vi "RealSense_HelloWorld_PointCloud.vi"() -> ()   [LabVIEW 2016]
doc: "Simple Demo showing how to connect a RealSense Camera to stream COLOR and DEPTH from the stereo camera of a D4xx series camera."
uses:
  <vilib>/Utility/miscctls.llb/LV3DPointTypeDef.ctl
  <vilib>/Utility/miscctls.llb/LVRGBAColorTypeDef.ctl
  <vilib>/picture/3D Picture Control/Object/Create Object (name).vi
  libRealSense3.lvlib
  <vilib>/picture/3D Picture Control/NI_3D Picture Control.lvlib
panel:
  in  "Display tab":T1(tab)
  out "Found \nRealSense":bool=TRUE
  out "height":i32=720
  out "width":i32=1280
  out "init results":T2={"camera name"="Intel RealSense 415", "camera S/N"="725112060291", "F/W"="05.08.08.00", "Sensor name"="Stereo Module", "api_version"=20801, "rscontext"=1827613840, "device_list"=610165840, "device count"=2, "Dev out"=1824884112, "sensor_list"=1824885136, "sensor count"=2, "Sensor out"=609327328}
  in  "Select Resolution":u16(ring)=27 items=["424 x 240 @6fps", "424 x 240 @15fps", "424 x 240 @30fps", "424 x 240 @60fps", "424 x 240 @90fps", "480 x 270 @6fps", "480 x 270 @15fps", "480 x 270 @30fps", "480 x 270 @60fps", "480 x 270 @90fps", "640 x 360 @6fps", "640 x 360 @15fps", "640 x 360 @30fps", "640 x 360 @60fps", "640 x 360 @90fps", "640 x 480 @6fps", "640 x 480 @15fps", "640 x 480 @30fps", "640 x 480 @60fps", "640 x 480 @90fps", "848 x 480 @6fps", "848 x 480 @15fps", "848 x 480 @30fps", "848 x 480 @60fps", "848 x 480 @90fps", "1280 x 720 @6fps", "1280 x 720 @15fps", "1280 x 720 @30fps"]
  in  "Sensor index":i32
  in  "Device index":i32
  out "L-R Baseline, mm":sgl=54.83181
  out "fy":sgl=952.6064 format="%#_5g"
  out "fx":sgl=952.6064 format="%#_5g"
  out "ppy":sgl=370.69974 format="%#_5g"
  out "ppx":sgl=634.5728 format="%#_5g"
  in  "Exposure,us":sgl=33000.0
  in  "Autoexposure":bool=TRUE
  in  "Depth Presets":T3(ring)=enum."Face2"
  in  "Color Presets":T4(ring)=enum."DS410 (DS5a) 4"
  in  "Laser on/off":bool=TRUE
  in  "Gain(16-248)":sgl=16.0 min=16 max=248
  in  "Update Presets":bool
  in  "Laser \nPower (mW)":dbl(slide)=155.72448 min=0.0 max=360.0 scale=0.36..360.0
  in  "Range Scale":enum16{"200m", "100m", "60m", "6m", "2m", "1m"}(ring)=enum."6m"
  out "RGB image":picture
  out "Depth map":sgl[][](graph)
  out "3D Picture":refnum<vi>(3d-picture)
  out "init error":string="No Error\rNo Error\rNo Error\rNo Error\rNo Error\rNo Error\rNo Error\rNo Error\rNo Error\rNo Error\rNo Error"
  out "Capture2 error":string="No Error"
  out "Start Error":string="No Error\rNo Error\rNo Error"
  out "Config error":string="No Error\rNo Error"
  out "Capture1 Error":string="No Error"
  out "Close Error":string="No Error\rNo Error\rNo Error\rNo Error"
  out "release frame error":string="No Error"
  out "iteration":i32=57
  in  "stop":bool=TRUE
  # "RealSense Hello World: PointCloud"
  # "This demo shows how to connect a RealSense D4xx Stereo Depth Camera, and display the textured PointCloud."
  # "Note; When you change Depth Preset you need to stop and restart for the HDAD settings to take effect.\n\nTry the Color preset called \"Remove IR2\". It will remove the laser projector from the RGB 1280x720 image."
  # "INTRINSICS & EXTRINSICS"
  # "SELECT THE RESOLUTION"
  # "DEPTH MAP"
  # "COLOR"
  # "Changes Color scale for Depth Map."
  # "20-1660000"
  # "3D POINTCLOUD"
  # "Rotate: Drag image\nMove X-Y: HOLD DOWN CTRL while dragging.\nZoom: SHIFT while dragging."
  # "ERRORS"
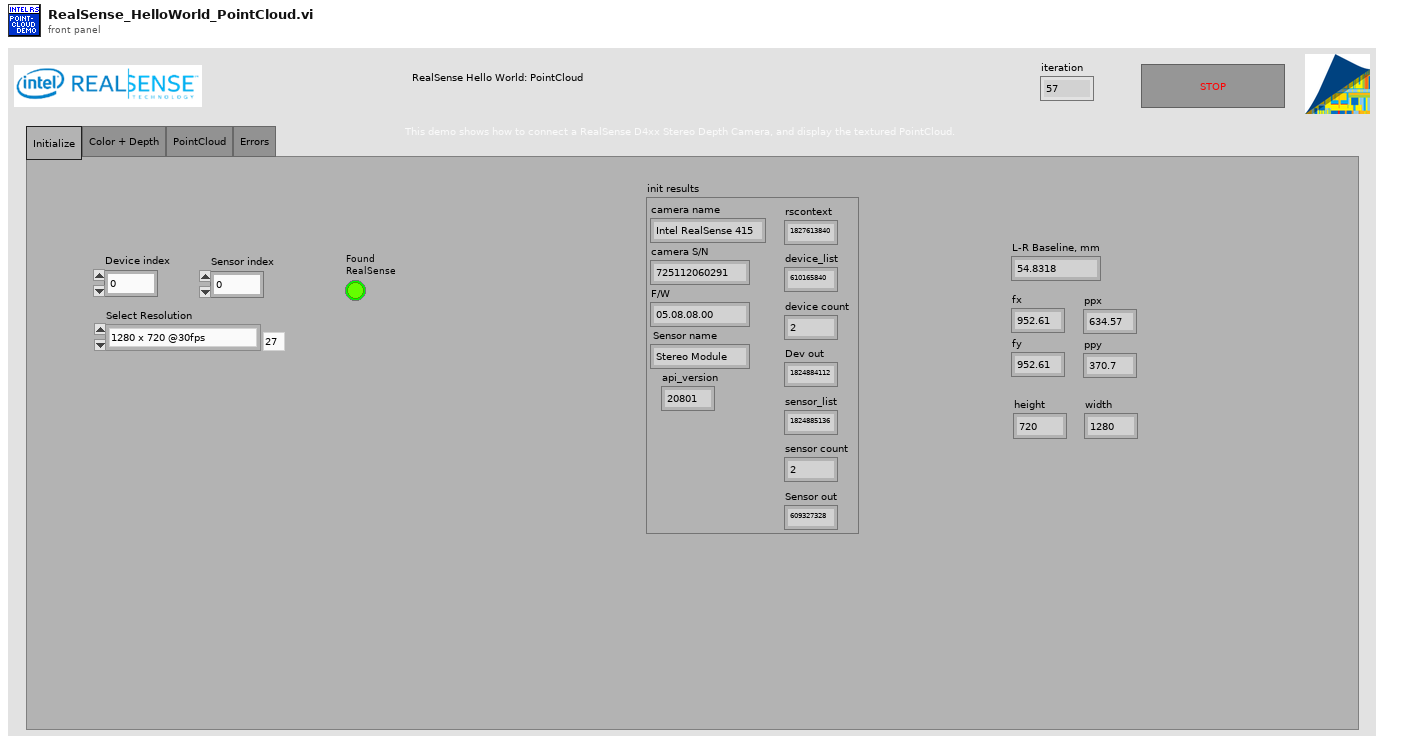
[diagram p1: front panel]
types:
  T1 = enum32{"Initialize", "Color + Depth", "PointCloud", "Errors"}
  T2 = cluster{"camera name":string, "camera S/N":string, "F/W":string, "Sensor name":string, "api_version":i32, "rscontext":u64, "device_list":u64, "device count":i32, "Dev out":u64, "sensor_list":u64, "sensor count":i32, "Sensor out":u64}
  T3 = enum16{"Custom", "Original", "New Depth 1", "New Depth 2", "Depth Active 1", "Active 3D Scan", "Active Short A", "Active Short C", "Face", "Face2", "Best Box", "High Density", "Medium Density", "High Accuracy", "Hand", "Short Range", "Flat wall", "Load .JSON", "Load .JSON2"}
  T4 = enum16{"Custom", "RS400 (DS5p)", "RS400 (DS5p) 2", "RS400 (DS5p) 3", "RS400 (DS5p) 4", "RS400 (DS5p) 5", "RS410 (DS5a)", "RS410 (DS5a) 2", "DS410 (DS5a) 3", "DS410 (DS5a) 4", "DS410+IR", "DS5LR", "DS5LR-2", "DS5LR no pattern", "RS410 Remove IR", "RS410 Remove IR 2", "DS5micro", "D435"}
  T5 = cluster{"width":i32, "height":i32, "fps":i32, "Profile":u64, "ppx":sgl, "ppy":sgl, "fx":sgl, "fy":sgl, "model":u32}
  T6 = enum16{"Overall", "Per Primitive", "Per Vertex", "Binding Off"}
  T7 = enum16{"Points", "Lines", "Line Strip", "Line Loop", "Triangles", "Triangle Strip", "Triangle Fan", "Quads", "Quad Strip", "Polygon"}
  T8 = enum16{"Depth", "Color (ext.)", "Color (left) ", "IR Left", "IR Right", "IR Left (Y16)", "IR Right (Y16)"}
  T9 = cluster{"R":dbl, "G":dbl, "B":dbl, "Alpha":dbl}[]
  T10 = typedef "LVRGBAColorTypeDef.ctl" = cluster{"Red":sgl, "Green":sgl, "Blue":sgl, "Alpha":sgl}
  T11 = typedef "LV3DPointTypeDef.ctl" = cluster{"X":sgl, "Y":sgl, "Z":sgl}
  T12 = cluster{"Alpha":sgl, "Blue":sgl, "Green":sgl, "Red":sgl}
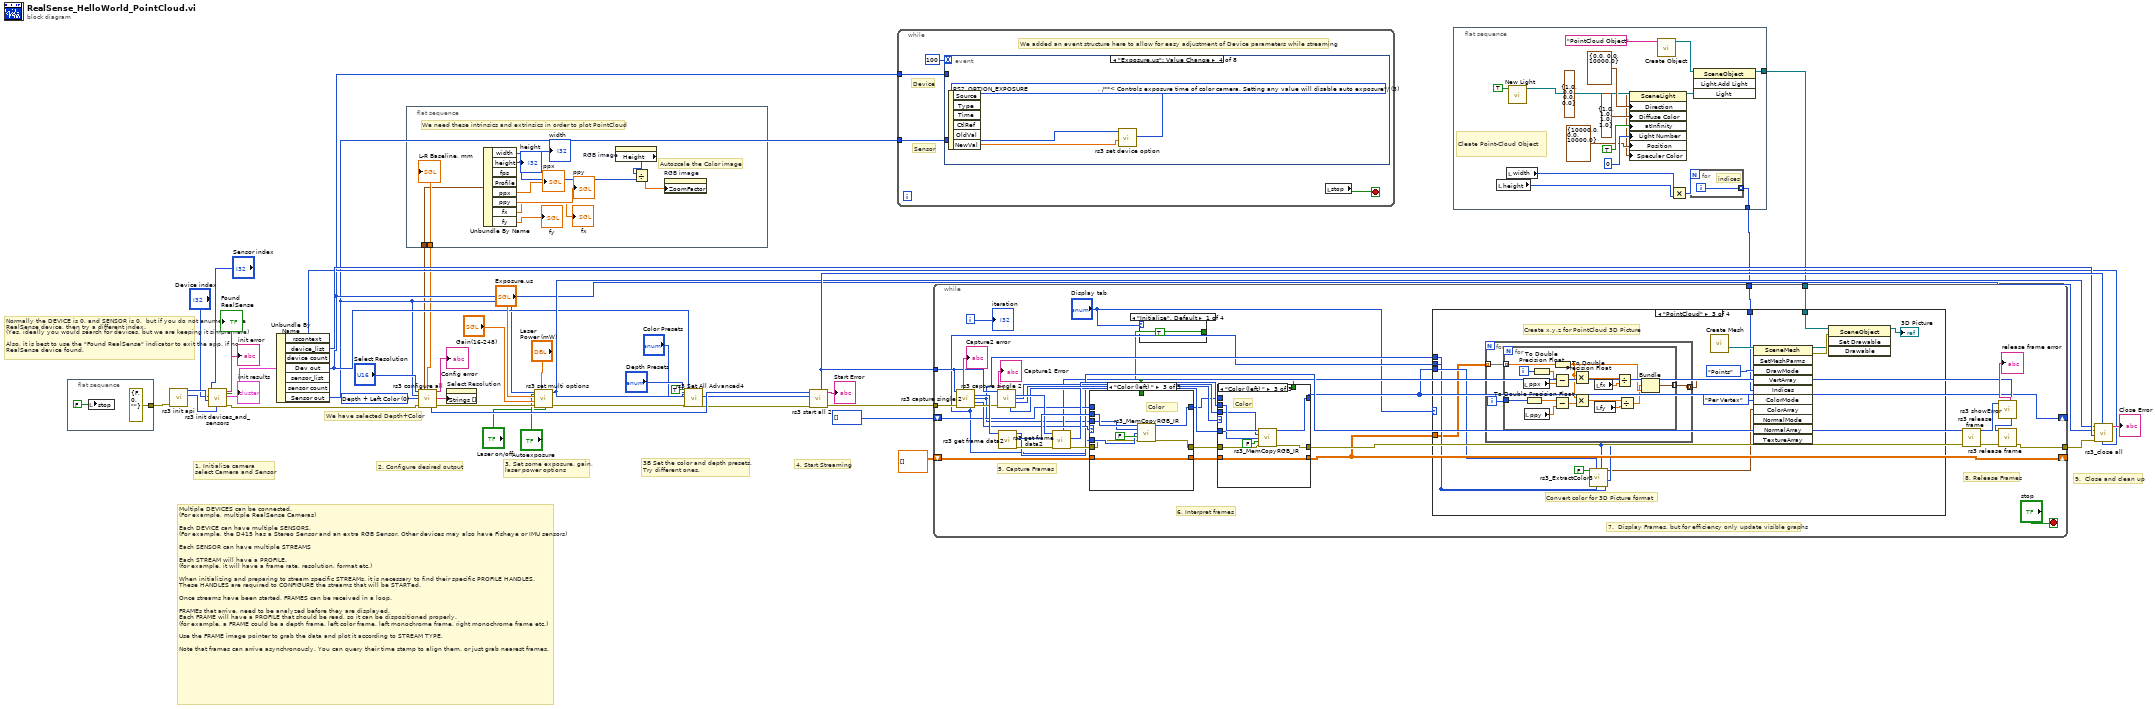
[diagram p0: block diagram]
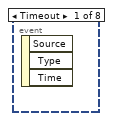
[diagram p2: hidden frame]
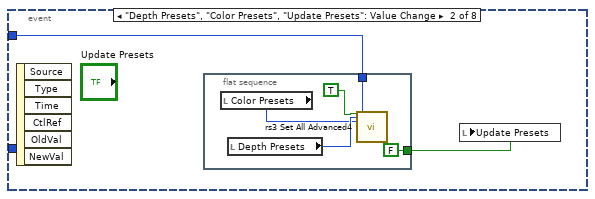
[diagram p3: hidden frame]
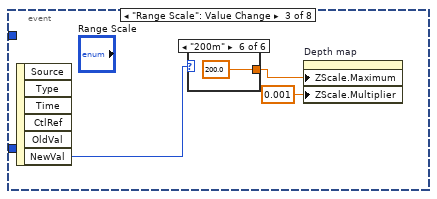
[diagram p4: hidden frame]
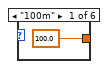
[diagram p5: hidden frame]
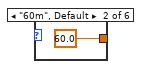
[diagram p6: hidden frame]
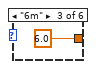
[diagram p7: hidden frame]
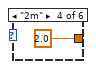
[diagram p8: hidden frame]
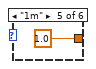
[diagram p9: hidden frame]
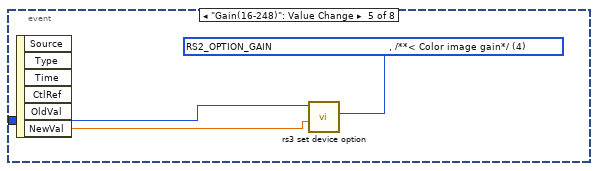
[diagram p10: hidden frame]
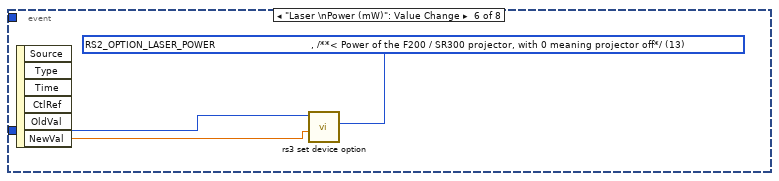
[diagram p11: hidden frame]
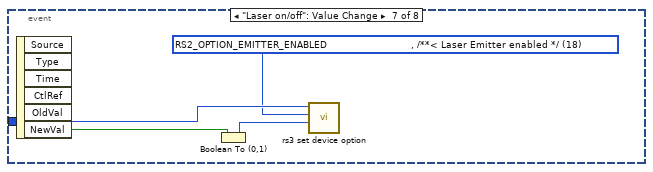
[diagram p12: hidden frame]
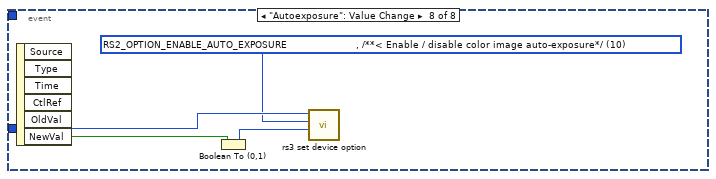
[diagram p13: hidden frame]
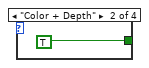
[diagram p14: hidden frame]
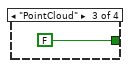
[diagram p15: hidden frame]
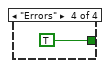
[diagram p16: hidden frame]
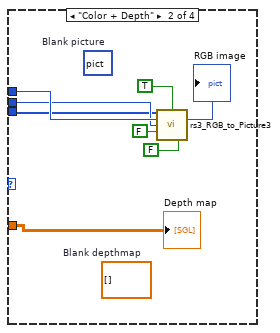
[diagram p18: hidden frame]
diagram:
  w29 = u16 0 items=["Depth + Left Color", "Unrectified L + R", "Rectified L + R"] ("Stream selection")
  # "3B Set the color and depth presets.\nTry different ones."
  # "We have selected Depth+Color"
  # "Normally the DEVICE is 0, and SENSOR is 0,  but if you do not enumerate the RealSense device, then try a different index.\n(Yes, ideally you would search for devices, but we are keeping it simple here)\n\nAlso, it is best to use the \"Found RealSense\" indicator to exit the app, if no RealSense device found."
  # "Multiple DEVICES can be connected. \n(For example, multiple RealSense Cameras)\n\nEach DEVICE can have multiple SENSORS. \n(For example, the D415 has a Stereo Sensor and an extra RGB Sensor. Other devices may also have Fisheye or IMU sensors) \n\nEach SENSOR can have multiple STREAMS\n\nEach STREAM will have a PROFILE. \n(for example, it will have a frame rate, resolution, format etc.)\n\nWhen initializing and preparing to stream specific STREAMs, it is necessary to find their specific PROFILE HANDLES.\nThese HANDLES are required to CONFIGURE the streams that will be STARTed. \n\nOnce streams have been started, FRAMES can be received in a loop. \n \nFRAMEs that arrive, need to be analyzed before they are displayed. \nEach FRAME will have a PROFILE that should be read, so it can be dispositioned properly.\n(for example, a FRAME could be a depth frame, left color frame, left monochrome frame, right monochrome frame etc.)\n\nUse the FRAME image pointer to grab the data and plot it according to STREAM TYPE.\n\nNote that frames can arrive asynchronously. You can query their time stamp to align them, or just grab nearest frames."
  # "9.  Close and clean up"
  # "4. Start Streaming"
  # "3. Set some exposure, gain, \nlaser power options"
  # "2. Configure desired output"
  # "1. Initialize camera\nselect Camera and Sensor"
  n1 = flat-sequence {
    tunnel: [errorcluster {"status"=FALSE, "code"=0, "source"=""} ("error in")] -> w30
    frame #0 {
      n2 = local write "stop"(FALSE ("stop")) -> ()
    }
  }
  n3 = call "rs3 init api.vi"("error in (no error)"=w30) -> ("rscontext"=w7:u64, "api_version"=w8:i32)  [unwired: 7 in, 2 out]
  n4 = call "rs3 init devices_and_sensors.vi"("rscontext"=w7, "api_version"=w8, "Select Device"="Device index", "Select Sensor"="Sensor index") -> ("error out"=w4:errorcluster, "init results"=w2:T2, "init error"=→"init error":string, "Found RealSense"=→"Found \nRealSense":bool)  [unwired: 1 in, 3 out]
  "init results" <- w2
  n5 = Unbundle By Name(w2) -> ("rscontext"=w35:u64, "device_list"=w36:u64, "Dev out"=w16:u64, "Sensor out"=w15:u64)  [unwired: 3 out]
  n6 = flat-sequence {
    tunnel: w13 -> [w53]
    tunnel: w12 -> [w52]
    frame #0 {
      # "Autoscale the Color image"
      # "We need these intrinsics and extrinsics in order to plot PointCloud"
      n7 = Unbundle By Name(w52) -> ("width"=→"width":i32, "height"=w50:i32, "ppx"=→"ppx":sgl, "ppy"=→"ppy":sgl, "fx"=→"fx":sgl, "fy"=→"fy":sgl)  [unwired: 2 out]
      "height" <- w50
      n8 = property on="RGB image" class="Pict"() -> ("Height"=w51:u32)  [unwired: 2 in, 2 out]
      n9 = Divide(x=w51, y=w50) -> (x/y=w49:dbl)
      n10 = property on="RGB image" class="Pict"("ZoomFactor"=w49) -> ()  [unwired: 2 in, 2 out]
      "L-R Baseline, mm" <- w53
    }
  }
  n11 = call "rs3 configure all.vi"("Select Resolution"="Select Resolution", "Sensor in"=w15, "Stream selection"=w29, "error in (no error)"=w4) -> ("Output stream L"=w12:T5, "config error"=→"Config error":string, "Output stream"=w31:string[], "L-R Baseline, mm"=w13:sgl, "Stream Profile Handles"=w41:u64[], "error out"=w28:errorcluster)  [unwired: 2 in, 4 out]
  n12 = property on="Select Resolution" class="Ring (strict)"("Strings []"=w31) -> ()  [unwired: 2 in, 2 out]
  n13 = call "rs3 set multi options.vi"("laser on/off"="Laser on/off", "autoexposure"="Autoexposure", "Laser power, mW (0-360)"="Laser \nPower (mW)", "error in (no error)"=w28, "Gain(16-248)"="Gain(16-248)", "Exposure, us"="Exposure,us", "Sensor in"=w15) -> ("error out"=w21:errorcluster, "Sensor out"=w27:u64)  [unwired: 2 in, 1 out]
  n14 = call "rs3 Set All Advanced4.vi"("Set Color Corr"=TRUE, "Depth Presets"="Depth Presets", "Color Presets"="Color Presets", "error in (no error)"=w21, "device in"=w16) -> ("error out"=w20:errorcluster)  [unwired: 20 in, 2 out]
  n15 = call "rs3 start all 2.vi"("error in (no error)"=w20, "Sensor in"=w27, "Stream profile array"=w41) -> ("error out"=w32:errorcluster, "Config Error"=→"Start Error":string, "queue out"=w40:u64)  [unwired: 5 in, 1 out]
  n16 = while {
    tunnel: w16 -> [w56]
    tunnel: w15 -> [w55]
    stop <- w57 stop-if-true
    # "Sensor"
    # "Device"
    # "We added an event structure here to allow for easy adjustment of Device parameters while streaming"
    n17 = event shown="[3] \"Exposure,us\": Value Change" {
      selector: _ -> [_ _ _ _ _ _ _ _]
      dyn-events: _ -> [_ _ _ _ _ _ _ _]
      timeout: 100 -> [_ _ _ _ _ _ _ _]
      tunnel: w56 -> [_ w59 _ _ _ _ _ _]
      tunnel: w55 -> [_ _ _ w76 w79 w82 w86 w90]
      event Timeout {
        n18 = event-data() -> ()  [unwired: 1 in, 3 out]
      }
      event "Depth Presets", "Color Presets", "Update Presets": Value Change {
        n19 = event-data() -> ()  [unwired: 1 in, 6 out]
        n20 = flat-sequence {
          tunnel: w59 -> [w61]
          tunnel: [FALSE ("Update Presets")] -> w58
          frame #0 {
            n21 = local read "Color Presets"() -> (w63:T4)
            n22 = local read "Depth Presets"() -> (w64:T3)
            n23 = call "rs3 Set All Advanced4.vi"("Set Color Corr"=TRUE, "Depth Presets"=w64, "Color Presets"=w63, "device in"=w61) -> ()  [unwired: 21 in, 3 out]
          }
        }
        n24 = local write "Update Presets"(w58) -> ()
      }
      event "Range Scale": Value Change {
        n25 = event-data() -> ("NewVal"=w66:enum16{"200m", "100m", "60m", "6m", "2m", "1m"})  [unwired: 1 in, 5 out]
        n26 = case shown="\"200m\"" w66 {
          tunnel: [100.0 ("Z Scale.Offset and Multiplier:Multiplier") 60.0 ("Z Scale.Offset and Multiplier:Multiplier") 6.0 ("Z Scale.Offset and Multiplier:Multiplier") 2.0 ("Z Scale.Offset and Multiplier:Multiplier") 1.0 ("Z Scale.Offset and Multiplier:Multiplier") 200.0 ("Z Scale.Offset and Multiplier:Multiplier")] -> w65
          frame "100m" {
          }
          frame "60m", Default {
          }
          frame "6m" {
          }
          frame "2m" {
          }
          frame "1m" {
          }
          frame "200m" {
          }
        }
        n27 = property on="Depth map" class="IntGraph (strict)"("ZScale.Maximum"=w65, "ZScale.Multiplier"=0.001 ("Z Scale.Offset and Multiplier:Multiplier")) -> ()  [unwired: 2 in, 2 out]
      }
      event "Exposure,us": Value Change {
        w74 = u16 3 items=["    RS2_OPTION_BACKLIGHT_COMPENSATION                     , /**< Enable / disable color backlight compensation*/", "    RS2_OPTION_BRIGHTNESS                                 , /**< Color image brightness*/", "    RS2_OPTION_CONTRAST                                   , /**< Color image contrast*/", "    RS2_OPTION_EXPOSURE                                   , /**< Controls exposure time of color camera. Setting any value will disable auto exposure*/", "    RS2_OPTION_GAIN                                       , /**< Color image gain*/", "    RS2_OPTION_GAMMA                                      , /**< Color image gamma setting*/", "    RS2_OPTION_HUE                                        , /**< Color image hue*/", "    RS2_OPTION_SATURATION                                 , /**< Color image saturation setting*/", "    RS2_OPTION_SHARPNESS                                  , /**< Color image sharpness setting*/", "    RS2_OPTION_WHITE_BALANCE                              , /**< Controls white balance of color image. Setting any value will disable auto white balance*/", "    RS2_OPTION_ENABLE_AUTO_EXPOSURE                       , /**< Enable / disable color image auto-exposure*/", "    RS2_OPTION_ENABLE_AUTO_WHITE_BALANCE                  , /**< Enable / disable color image auto-white-balance*/", "    RS2_OPTION_VISUAL_PRESET                              , /**< Provide access to several recommend sets of option presets for the depth camera */", "    RS2_OPTION_LASER_POWER                                , /**< Power of the F200 / SR300 projector, with 0 meaning projector off*/", "    RS2_OPTION_ACCURACY                                   , /**< Set the number of patterns projected per frame. The higher the accuracy value the more patterns projected. Increasing the number of patterns help to achieve better accuracy. Note that this c", "    RS2_OPTION_MOTION_RANGE                               , /**< Motion vs. Range trade-off, with lower values allowing for better motion sensitivity and higher values allowing for better depth range*/", "    RS2_OPTION_FILTER_OPTION                              , /**< Set the filter to apply to each depth frame. Each one of the filter is optimized per the application requirements*/", "    RS2_OPTION_CONFIDENCE_THRESHOLD                       , /**< The confidence level threshold used by the Depth algorithm pipe to set whether a pixel will get a valid range or will be marked with invalid range*/", "    RS2_OPTION_EMITTER_ENABLED                            , /**< Laser Emitter enabled */", "    RS2_OPTION_FRAMES_QUEUE_SIZE                          , /**< Number of frames the user is allowed to keep per stream. Trying to hold-on to more frames will cause frame-drops.*/", "    RS2_OPTION_TOTAL_FRAME_DROPS                          , /**< Total number of detected frame drops from all streams */", "    RS2_OPTION_AUTO_EXPOSURE_MODE                         , /**< Auto-Exposure modes: Static, Anti-Flicker and Hybrid */", "    RS2_OPTION_POWER_LINE_FREQUENCY                       , /**< Power Line Frequency control for anti-flickering Off/50Hz/60Hz/Auto */", "    RS2_OPTION_ASIC_TEMPERATURE                           , /**< Current Asic Temperature */", "    RS2_OPTION_ERROR_POLLING_ENABLED                      , /**< disable error handling */", "    RS2_OPTION_PROJECTOR_TEMPERATURE                      , /**< Current Projector Temperature */", "    RS2_OPTION_OUTPUT_TRIGGER_ENABLED                     , /**< Enable / disable trigger to be outputed from the camera to any external device on every depth frame */", "    RS2_OPTION_MOTION_MODULE_TEMPERATURE                  , /**< Current Motion-Module Temperature */", "    RS2_OPTION_DEPTH_UNITS                                , /**< Number of meters represented by a single depth unit */", "    RS2_OPTION_ENABLE_MOTION_CORRECTION                   , /**< Enable/Disable automatic correction of the motion data */", "    RS2_OPTION_AUTO_EXPOSURE_PRIORITY                     , /**< Allows sensor to dynamically ajust the frame rate depending on lighting conditions */", "    RS2_OPTION_COUNT                                      , /**< Number of enumeration values. Not a valid input: intended to be used in for-loops. */"] ("RS Option")
        n28 = event-data() -> ("NewVal"=w75:sgl)  [unwired: 1 in, 5 out]
        n29 = call "rs3 set device option.vi"("value"=w75, "RS Option"=w74, "Sensor in"=w76) -> ()  [unwired: 6 in, 3 out]
      }
      event "Gain(16-248)": Value Change {
        w77 = u16 4 items=["    RS2_OPTION_BACKLIGHT_COMPENSATION                     , /**< Enable / disable color backlight compensation*/", "    RS2_OPTION_BRIGHTNESS                                 , /**< Color image brightness*/", "    RS2_OPTION_CONTRAST                                   , /**< Color image contrast*/", "    RS2_OPTION_EXPOSURE                                   , /**< Controls exposure time of color camera. Setting any value will disable auto exposure*/", "    RS2_OPTION_GAIN                                       , /**< Color image gain*/", "    RS2_OPTION_GAMMA                                      , /**< Color image gamma setting*/", "    RS2_OPTION_HUE                                        , /**< Color image hue*/", "    RS2_OPTION_SATURATION                                 , /**< Color image saturation setting*/", "    RS2_OPTION_SHARPNESS                                  , /**< Color image sharpness setting*/", "    RS2_OPTION_WHITE_BALANCE                              , /**< Controls white balance of color image. Setting any value will disable auto white balance*/", "    RS2_OPTION_ENABLE_AUTO_EXPOSURE                       , /**< Enable / disable color image auto-exposure*/", "    RS2_OPTION_ENABLE_AUTO_WHITE_BALANCE                  , /**< Enable / disable color image auto-white-balance*/", "    RS2_OPTION_VISUAL_PRESET                              , /**< Provide access to several recommend sets of option presets for the depth camera */", "    RS2_OPTION_LASER_POWER                                , /**< Power of the F200 / SR300 projector, with 0 meaning projector off*/", "    RS2_OPTION_ACCURACY                                   , /**< Set the number of patterns projected per frame. The higher the accuracy value the more patterns projected. Increasing the number of patterns help to achieve better accuracy. Note that this c", "    RS2_OPTION_MOTION_RANGE                               , /**< Motion vs. Range trade-off, with lower values allowing for better motion sensitivity and higher values allowing for better depth range*/", "    RS2_OPTION_FILTER_OPTION                              , /**< Set the filter to apply to each depth frame. Each one of the filter is optimized per the application requirements*/", "    RS2_OPTION_CONFIDENCE_THRESHOLD                       , /**< The confidence level threshold used by the Depth algorithm pipe to set whether a pixel will get a valid range or will be marked with invalid range*/", "    RS2_OPTION_EMITTER_ENABLED                            , /**< Laser Emitter enabled */", "    RS2_OPTION_FRAMES_QUEUE_SIZE                          , /**< Number of frames the user is allowed to keep per stream. Trying to hold-on to more frames will cause frame-drops.*/", "    RS2_OPTION_TOTAL_FRAME_DROPS                          , /**< Total number of detected frame drops from all streams */", "    RS2_OPTION_AUTO_EXPOSURE_MODE                         , /**< Auto-Exposure modes: Static, Anti-Flicker and Hybrid */", "    RS2_OPTION_POWER_LINE_FREQUENCY                       , /**< Power Line Frequency control for anti-flickering Off/50Hz/60Hz/Auto */", "    RS2_OPTION_ASIC_TEMPERATURE                           , /**< Current Asic Temperature */", "    RS2_OPTION_ERROR_POLLING_ENABLED                      , /**< disable error handling */", "    RS2_OPTION_PROJECTOR_TEMPERATURE                      , /**< Current Projector Temperature */", "    RS2_OPTION_OUTPUT_TRIGGER_ENABLED                     , /**< Enable / disable trigger to be outputed from the camera to any external device on every depth frame */", "    RS2_OPTION_MOTION_MODULE_TEMPERATURE                  , /**< Current Motion-Module Temperature */", "    RS2_OPTION_DEPTH_UNITS                                , /**< Number of meters represented by a single depth unit */", "    RS2_OPTION_ENABLE_MOTION_CORRECTION                   , /**< Enable/Disable automatic correction of the motion data */", "    RS2_OPTION_AUTO_EXPOSURE_PRIORITY                     , /**< Allows sensor to dynamically ajust the frame rate depending on lighting conditions */", "    RS2_OPTION_COUNT                                      , /**< Number of enumeration values. Not a valid input: intended to be used in for-loops. */"] ("RS Option")
        n30 = event-data() -> ("NewVal"=w78:sgl)  [unwired: 1 in, 5 out]
        n31 = call "rs3 set device option.vi"("value"=w78, "RS Option"=w77, "Sensor in"=w79) -> ()  [unwired: 6 in, 3 out]
      }
      event "Laser \nPower (mW)": Value Change {
        w80 = u16 13 items=["    RS2_OPTION_BACKLIGHT_COMPENSATION                     , /**< Enable / disable color backlight compensation*/", "    RS2_OPTION_BRIGHTNESS                                 , /**< Color image brightness*/", "    RS2_OPTION_CONTRAST                                   , /**< Color image contrast*/", "    RS2_OPTION_EXPOSURE                                   , /**< Controls exposure time of color camera. Setting any value will disable auto exposure*/", "    RS2_OPTION_GAIN                                       , /**< Color image gain*/", "    RS2_OPTION_GAMMA                                      , /**< Color image gamma setting*/", "    RS2_OPTION_HUE                                        , /**< Color image hue*/", "    RS2_OPTION_SATURATION                                 , /**< Color image saturation setting*/", "    RS2_OPTION_SHARPNESS                                  , /**< Color image sharpness setting*/", "    RS2_OPTION_WHITE_BALANCE                              , /**< Controls white balance of color image. Setting any value will disable auto white balance*/", "    RS2_OPTION_ENABLE_AUTO_EXPOSURE                       , /**< Enable / disable color image auto-exposure*/", "    RS2_OPTION_ENABLE_AUTO_WHITE_BALANCE                  , /**< Enable / disable color image auto-white-balance*/", "    RS2_OPTION_VISUAL_PRESET                              , /**< Provide access to several recommend sets of option presets for the depth camera */", "    RS2_OPTION_LASER_POWER                                , /**< Power of the F200 / SR300 projector, with 0 meaning projector off*/", "    RS2_OPTION_ACCURACY                                   , /**< Set the number of patterns projected per frame. The higher the accuracy value the more patterns projected. Increasing the number of patterns help to achieve better accuracy. Note that this c", "    RS2_OPTION_MOTION_RANGE                               , /**< Motion vs. Range trade-off, with lower values allowing for better motion sensitivity and higher values allowing for better depth range*/", "    RS2_OPTION_FILTER_OPTION                              , /**< Set the filter to apply to each depth frame. Each one of the filter is optimized per the application requirements*/", "    RS2_OPTION_CONFIDENCE_THRESHOLD                       , /**< The confidence level threshold used by the Depth algorithm pipe to set whether a pixel will get a valid range or will be marked with invalid range*/", "    RS2_OPTION_EMITTER_ENABLED                            , /**< Laser Emitter enabled */", "    RS2_OPTION_FRAMES_QUEUE_SIZE                          , /**< Number of frames the user is allowed to keep per stream. Trying to hold-on to more frames will cause frame-drops.*/", "    RS2_OPTION_TOTAL_FRAME_DROPS                          , /**< Total number of detected frame drops from all streams */", "    RS2_OPTION_AUTO_EXPOSURE_MODE                         , /**< Auto-Exposure modes: Static, Anti-Flicker and Hybrid */", "    RS2_OPTION_POWER_LINE_FREQUENCY                       , /**< Power Line Frequency control for anti-flickering Off/50Hz/60Hz/Auto */", "    RS2_OPTION_ASIC_TEMPERATURE                           , /**< Current Asic Temperature */", "    RS2_OPTION_ERROR_POLLING_ENABLED                      , /**< disable error handling */", "    RS2_OPTION_PROJECTOR_TEMPERATURE                      , /**< Current Projector Temperature */", "    RS2_OPTION_OUTPUT_TRIGGER_ENABLED                     , /**< Enable / disable trigger to be outputed from the camera to any external device on every depth frame */", "    RS2_OPTION_MOTION_MODULE_TEMPERATURE                  , /**< Current Motion-Module Temperature */", "    RS2_OPTION_DEPTH_UNITS                                , /**< Number of meters represented by a single depth unit */", "    RS2_OPTION_ENABLE_MOTION_CORRECTION                   , /**< Enable/Disable automatic correction of the motion data */", "    RS2_OPTION_AUTO_EXPOSURE_PRIORITY                     , /**< Allows sensor to dynamically ajust the frame rate depending on lighting conditions */", "    RS2_OPTION_COUNT                                      , /**< Number of enumeration values. Not a valid input: intended to be used in for-loops. */"] ("RS Option")
        n32 = event-data() -> ("NewVal"=w81:dbl)  [unwired: 1 in, 5 out]
        n33 = call "rs3 set device option.vi"("value"=w81, "RS Option"=w80, "Sensor in"=w82) -> ()  [unwired: 6 in, 3 out]
      }
      event "Laser on/off": Value Change {
        w85 = u16 18 items=["    RS2_OPTION_BACKLIGHT_COMPENSATION                     , /**< Enable / disable color backlight compensation*/", "    RS2_OPTION_BRIGHTNESS                                 , /**< Color image brightness*/", "    RS2_OPTION_CONTRAST                                   , /**< Color image contrast*/", "    RS2_OPTION_EXPOSURE                                   , /**< Controls exposure time of color camera. Setting any value will disable auto exposure*/", "    RS2_OPTION_GAIN                                       , /**< Color image gain*/", "    RS2_OPTION_GAMMA                                      , /**< Color image gamma setting*/", "    RS2_OPTION_HUE                                        , /**< Color image hue*/", "    RS2_OPTION_SATURATION                                 , /**< Color image saturation setting*/", "    RS2_OPTION_SHARPNESS                                  , /**< Color image sharpness setting*/", "    RS2_OPTION_WHITE_BALANCE                              , /**< Controls white balance of color image. Setting any value will disable auto white balance*/", "    RS2_OPTION_ENABLE_AUTO_EXPOSURE                       , /**< Enable / disable color image auto-exposure*/", "    RS2_OPTION_ENABLE_AUTO_WHITE_BALANCE                  , /**< Enable / disable color image auto-white-balance*/", "    RS2_OPTION_VISUAL_PRESET                              , /**< Provide access to several recommend sets of option presets for the depth camera */", "    RS2_OPTION_LASER_POWER                                , /**< Power of the F200 / SR300 projector, with 0 meaning projector off*/", "    RS2_OPTION_ACCURACY                                   , /**< Set the number of patterns projected per frame. The higher the accuracy value the more patterns projected. Increasing the number of patterns help to achieve better accuracy. Note that this c", "    RS2_OPTION_MOTION_RANGE                               , /**< Motion vs. Range trade-off, with lower values allowing for better motion sensitivity and higher values allowing for better depth range*/", "    RS2_OPTION_FILTER_OPTION                              , /**< Set the filter to apply to each depth frame. Each one of the filter is optimized per the application requirements*/", "    RS2_OPTION_CONFIDENCE_THRESHOLD                       , /**< The confidence level threshold used by the Depth algorithm pipe to set whether a pixel will get a valid range or will be marked with invalid range*/", "    RS2_OPTION_EMITTER_ENABLED                            , /**< Laser Emitter enabled */", "    RS2_OPTION_FRAMES_QUEUE_SIZE                          , /**< Number of frames the user is allowed to keep per stream. Trying to hold-on to more frames will cause frame-drops.*/", "    RS2_OPTION_TOTAL_FRAME_DROPS                          , /**< Total number of detected frame drops from all streams */", "    RS2_OPTION_AUTO_EXPOSURE_MODE                         , /**< Auto-Exposure modes: Static, Anti-Flicker and Hybrid */", "    RS2_OPTION_POWER_LINE_FREQUENCY                       , /**< Power Line Frequency control for anti-flickering Off/50Hz/60Hz/Auto */", "    RS2_OPTION_ASIC_TEMPERATURE                           , /**< Current Asic Temperature */", "    RS2_OPTION_ERROR_POLLING_ENABLED                      , /**< disable error handling */", "    RS2_OPTION_PROJECTOR_TEMPERATURE                      , /**< Current Projector Temperature */", "    RS2_OPTION_OUTPUT_TRIGGER_ENABLED                     , /**< Enable / disable trigger to be outputed from the camera to any external device on every depth frame */", "    RS2_OPTION_MOTION_MODULE_TEMPERATURE                  , /**< Current Motion-Module Temperature */", "    RS2_OPTION_DEPTH_UNITS                                , /**< Number of meters represented by a single depth unit */", "    RS2_OPTION_ENABLE_MOTION_CORRECTION                   , /**< Enable/Disable automatic correction of the motion data */", "    RS2_OPTION_AUTO_EXPOSURE_PRIORITY                     , /**< Allows sensor to dynamically ajust the frame rate depending on lighting conditions */", "    RS2_OPTION_COUNT                                      , /**< Number of enumeration values. Not a valid input: intended to be used in for-loops. */"] ("RS Option")
        n34 = event-data() -> ("NewVal"=w84:bool)  [unwired: 1 in, 5 out]
        n35 = Boolean To (0,1)(Boolean=w84) -> (0, 1=w83:i16)
        n36 = call "rs3 set device option.vi"("value"=w83, "RS Option"=w85, "Sensor in"=w86) -> ()  [unwired: 6 in, 3 out]
      }
      event "Autoexposure": Value Change {
        w89 = u16 10 items=["    RS2_OPTION_BACKLIGHT_COMPENSATION                     , /**< Enable / disable color backlight compensation*/", "    RS2_OPTION_BRIGHTNESS                                 , /**< Color image brightness*/", "    RS2_OPTION_CONTRAST                                   , /**< Color image contrast*/", "    RS2_OPTION_EXPOSURE                                   , /**< Controls exposure time of color camera. Setting any value will disable auto exposure*/", "    RS2_OPTION_GAIN                                       , /**< Color image gain*/", "    RS2_OPTION_GAMMA                                      , /**< Color image gamma setting*/", "    RS2_OPTION_HUE                                        , /**< Color image hue*/", "    RS2_OPTION_SATURATION                                 , /**< Color image saturation setting*/", "    RS2_OPTION_SHARPNESS                                  , /**< Color image sharpness setting*/", "    RS2_OPTION_WHITE_BALANCE                              , /**< Controls white balance of color image. Setting any value will disable auto white balance*/", "    RS2_OPTION_ENABLE_AUTO_EXPOSURE                       , /**< Enable / disable color image auto-exposure*/", "    RS2_OPTION_ENABLE_AUTO_WHITE_BALANCE                  , /**< Enable / disable color image auto-white-balance*/", "    RS2_OPTION_VISUAL_PRESET                              , /**< Provide access to several recommend sets of option presets for the depth camera */", "    RS2_OPTION_LASER_POWER                                , /**< Power of the F200 / SR300 projector, with 0 meaning projector off*/", "    RS2_OPTION_ACCURACY                                   , /**< Set the number of patterns projected per frame. The higher the accuracy value the more patterns projected. Increasing the number of patterns help to achieve better accuracy. Note that this c", "    RS2_OPTION_MOTION_RANGE                               , /**< Motion vs. Range trade-off, with lower values allowing for better motion sensitivity and higher values allowing for better depth range*/", "    RS2_OPTION_FILTER_OPTION                              , /**< Set the filter to apply to each depth frame. Each one of the filter is optimized per the application requirements*/", "    RS2_OPTION_CONFIDENCE_THRESHOLD                       , /**< The confidence level threshold used by the Depth algorithm pipe to set whether a pixel will get a valid range or will be marked with invalid range*/", "    RS2_OPTION_EMITTER_ENABLED                            , /**< Laser Emitter enabled */", "    RS2_OPTION_FRAMES_QUEUE_SIZE                          , /**< Number of frames the user is allowed to keep per stream. Trying to hold-on to more frames will cause frame-drops.*/", "    RS2_OPTION_TOTAL_FRAME_DROPS                          , /**< Total number of detected frame drops from all streams */", "    RS2_OPTION_AUTO_EXPOSURE_MODE                         , /**< Auto-Exposure modes: Static, Anti-Flicker and Hybrid */", "    RS2_OPTION_POWER_LINE_FREQUENCY                       , /**< Power Line Frequency control for anti-flickering Off/50Hz/60Hz/Auto */", "    RS2_OPTION_ASIC_TEMPERATURE                           , /**< Current Asic Temperature */", "    RS2_OPTION_ERROR_POLLING_ENABLED                      , /**< disable error handling */", "    RS2_OPTION_PROJECTOR_TEMPERATURE                      , /**< Current Projector Temperature */", "    RS2_OPTION_OUTPUT_TRIGGER_ENABLED                     , /**< Enable / disable trigger to be outputed from the camera to any external device on every depth frame */", "    RS2_OPTION_MOTION_MODULE_TEMPERATURE                  , /**< Current Motion-Module Temperature */", "    RS2_OPTION_DEPTH_UNITS                                , /**< Number of meters represented by a single depth unit */", "    RS2_OPTION_ENABLE_MOTION_CORRECTION                   , /**< Enable/Disable automatic correction of the motion data */", "    RS2_OPTION_AUTO_EXPOSURE_PRIORITY                     , /**< Allows sensor to dynamically ajust the frame rate depending on lighting conditions */", "    RS2_OPTION_COUNT                                      , /**< Number of enumeration values. Not a valid input: intended to be used in for-loops. */"] ("RS Option")
        n37 = event-data() -> ("NewVal"=w88:bool)  [unwired: 1 in, 5 out]
        n38 = Boolean To (0,1)(Boolean=w88) -> (0, 1=w87:i16)
        n39 = call "rs3 set device option.vi"("value"=w87, "RS Option"=w89, "Sensor in"=w90) -> ()  [unwired: 6 in, 3 out]
      }
    }
    n40 = local read "stop"() -> (w57:bool)
  }
  n41 = while {
    tunnel: w40 -> [w117]
    tunnel: w32 -> [w127]
    tunnel: [w122] -> w39
    shift-right: [w96] -> _
    shift-left: sgl[][] [] ("2D Array Output") -> [w104]
    shift-right: [w98] -> _
    shift-left: u8[] [] ("Output Array") -> [w102]
    tunnel: w11 -> [w94]
    tunnel: w10 -> [w93]
    i -> [w126]
    stop <- "stop" stop-if-true
    # "8. Release Frames"
    # "7.  Display Frames, but for efficiency only update visible graphs"
    # "6. Interpret frames"
    # "5. Capture Frames"
    n42 = call "rs3 capture single 2.vi"("queue in"=w117, "error in (no error)"=w127) -> ("Capture Error"=→"Capture2 error":string, "frame out"=w125:u64, "width"=w97:i32, "Stream type"=w105:T8, "height"=w95:i32, "error out"=w118:errorcluster)  [unwired: 3 in, 5 out]
    n43 = call "rs3 capture single 2.vi"("queue in"=w117, "error in (no error)"=w118) -> ("Capture Error"=→"Capture1 Error":string, "frame out"=w115:u64, "width"=w107:i32, "Stream type"=w109:T8, "height"=w106:i32)  [unwired: 3 in, 6 out]
    n44 = call "rs3 get frame data2.vi"("frame in"=w125) -> ("error out"=w121:errorcluster, "image pointer out"=w124:u64, "Frame out"=w100:u64)  [unwired: 7 in, 1 out]
    n45 = call "rs3 get frame data2.vi"("error in (no error)"=w121, "frame in"=w115) -> ("error out"=w120:errorcluster, "image pointer out"=w108:u64, "Frame out"=w99:u64)  [unwired: 6 in, 1 out]
    n46 = case shown="\"Initialize\", Default" "Display tab" {
      tunnel: [TRUE ("Transpose") TRUE ("Transpose") FALSE ("Transpose") TRUE ("Transpose")] -> w91
      frame "Initialize", Default {
      }
      frame "Color + Depth" {
      }
      frame "PointCloud" {
      }
      frame "Errors" {
      }
    }
    n47 = case shown="\"Color (left) \"" w105 {
      tunnel: [w197 w203 w210] -> w111
      tunnel: w124 -> [_ w201 w213]
      tunnel: w97 -> [_ w200 w212]
      tunnel: w95 -> [_ w199 w211]
      tunnel: w120 -> [w197 w204 w209]
      tunnel: [w196 w205 w207] -> w103
      tunnel: w104 -> [w196 _ w207]
      tunnel: w102 -> [w195 w202 _]
      tunnel: [w195 w202 w208] -> w101
      tunnel: w91 -> [_ w198 _]
      frame "Color (ext.)", Default {
      }
      frame "Depth" {
        w206 = u16 0 items=["Y16", "Y8"] ("Image format")
        # "Depth"
        n48 = call "rs3_MemCopyUINT16_3.vi"("Image format"=w206, "Transpose"=w198, "error in (no error)"=w204, "Depth Y"=w199, "Depth X"=w200, "Zimage pointer"=w201) -> ("error out"=w203:errorcluster, "2D Array Output"=w205:sgl[][])  [unwired: 2 in, 2 out]
      }
      frame "Color (left) " {
        # "Color"
        n49 = call "rs3_MemCopyRGB_IR.vi"("Zimage pointer"=w213, "RGB  X, width"=w212, "RGB Y, height"=w211, "Monochrome(T)/Color(F)"=FALSE ("Grey(T)/Color(F)"), "error in (no error)"=w209) -> ("Output Array"=w208:u8[], "error out"=w210:errorcluster)  [unwired: 8 in, 1 out]
      }
    }
    n50 = case shown="\"Color (left) \"" w109 {
      tunnel: [w177 w183 w192] -> w110
      tunnel: w108 -> [_ w180 w191]
      tunnel: w107 -> [_ w179 w190]
      tunnel: w106 -> [_ w181 w189]
      tunnel: w111 -> [w177 w184 w193]
      tunnel: w103 -> [w176 _ w187]
      tunnel: [w176 w185 w187] -> w96
      tunnel: [w175 w186 w188] -> w98
      tunnel: w101 -> [w175 w186 _]
      tunnel: w91 -> [_ w178 _]
      frame "Color (ext.)", Default {
      }
      frame "Depth" {
        w182 = u16 0 items=["Y16", "Y8"] ("Image format")
        # "Depth"
        n51 = call "rs3_MemCopyUINT16_3.vi"("Image format"=w182, "Transpose"=w178, "error in (no error)"=w184, "Depth Y"=w181, "Depth X"=w179, "Zimage pointer"=w180) -> ("error out"=w183:errorcluster, "2D Array Output"=w185:sgl[][])  [unwired: 2 in, 2 out]
      }
      frame "Color (left) " {
        # "Color"
        n52 = call "rs3_MemCopyRGB_IR.vi"("Zimage pointer"=w191, "RGB  X, width"=w190, "RGB Y, height"=w189, "Monochrome(T)/Color(F)"=FALSE ("Grey(T)/Color(F)"), "error in (no error)"=w193) -> ("Output Array"=w188:u8[], "error out"=w192:errorcluster)  [unwired: 8 in, 1 out]
      }
    }
    n53 = case shown="\"PointCloud\"" "Display tab" {
      tunnel: w98 -> [_ w134 w154 _]
      tunnel: w97 -> [_ w136 w153 _]
      tunnel: w95 -> [_ w135 w152 _]
      tunnel: w96 -> [_ w133 w140 _]
      tunnel: w94 -> [_ _ w142 _]
      tunnel: w93 -> [_ _ w141 _]
      frame "Initialize", Default {
      }
      frame "Color + Depth" {
        (unwired) sgl[][] []  # Blank depthmap
        (unwired) picture bytes[33]  # Blank picture
        n54 = call "rs3_RGB_to_Picture3.vi"("RGB array"=w134, "Color(T)/Greyscale(F)"=TRUE, "RGB  X, width"=w136, "RGB Y, height"=w135, "AWB"=FALSE, "White Balance"=FALSE) -> ("new picture"=→"RGB image":picture)  [unwired: 8 in, 1 out]
        "Depth map" <- w133
      }
      frame "PointCloud" {
        # "Convert color for 3D Picture format"
        # "Create x,y,z for PointCloud 3D Picture"
        n55 = for {
          tunnel: w140 -> [w157] mode=indexing
          tunnel: [w156] -> w146 mode=concatenating
          i -> [w155]
          n56 = for {
            tunnel: w157 -> [w174] mode=indexing
            tunnel: w155 -> [w173]
            tunnel: [w172] -> w156 mode=indexing
            i -> [w171]
            n57 = local read "ppx"() -> (w164:sgl)
            n58 = local read "ppy"() -> (w162:sgl)
            n59 = To Double Precision Float(number=w173) -> (double precision float=w161:dbl)
            n60 = To Double Precision Float(number=w171) -> (double precision float=w166:dbl)
            n61 = Subtract(x=w166, y=w164) -> (x-y=w165:dbl)
            n62 = Subtract(x=w161, y=w162) -> (x-y=w160:dbl)
            n63 = To Double Precision Float(number=w174) -> (double precision float=w159:dbl)
            n64 = Multiply(x=w159, y=w165) -> (x*y=w170:dbl)
            n65 = Multiply(x=w159, y=w160) -> (x*y=w167:dbl)
            n66 = local read "fx"() -> (w169:sgl)
            n67 = local read "fy"() -> (w163:sgl)
            n68 = Divide(x=w170, y=w169) -> (x/y=w168:dbl)
            n69 = Divide(x=w167, y=w163) -> (x/y=w158:dbl)
            n70 = Bundle(w168, w158, w159) -> (w172:cluster{dbl, dbl, dbl})  [unwired: 1 in]
          }
        }
        n71 = call "rs3_ExtractColor3.vi"("Depth X"=w153, "Depth Y"=w152, "RGB Y"=w152, "RGB  X"=w153, "24bit Color Array"=w154, "White Balance"=FALSE) -> ("Norm Mesh Color"=w145:T9)  [unwired: 5 in]
        n72 = call <vilib>:"Create Mesh.vi"() -> ("New Mesh Refnum"=w148:refnum<vi>)  [unwired: 10 in, 1 out]
        n73 = invoke class="SceneMesh" method="SetMeshParms"(reference=w148, "DrawMode"=T7."Points" ("Draw Mode"), "VertArray"=w146, "Indices"=w141, "ColorMode"=T6."Per Vertex" ("Color Binding Mode"), "ColorArray"=w145) -> (reference out=w149:refnum<vi>, error out=w150:errorcluster)  [unwired: 5 in, 9 out]
        n74 = invoke class="SceneObject" method="Set Drawable"(reference=w142, error in=w150, "Drawable"=w149) -> (reference out=→"3D Picture":refnum<vi>)  [unwired: 1 in, 3 out]
      }
      frame "Errors" {
      }
    }
    n75 = call "rs3 release frame.vi"("error in (no error)"=w110, "Frame"=w100) -> ("error out"=w123:errorcluster, "error"=w114:u64)  [unwired: 8 in]
    n76 = call "rs3 showError.vi"("error"=w114) -> ("Error summary"=→"release frame error":string)  [unwired: 6 in, 4 out]
    n77 = call "rs3 release frame.vi"("error in (no error)"=w123, "Frame"=w99) -> ("error out"=w122:errorcluster)  [unwired: 8 in, 1 out]
    "iteration" <- w126
  }
  n78 = flat-sequence {
    tunnel: [w219] -> w11
    tunnel: [w215] -> w10
    frame #0 {
      # "Cleate Point-Cloud Object"
      n79 = local read "height"() -> (w216:i32)
      n80 = local read "width"() -> (w217:i32)
      n81 = call <vilib>:"New Light.vi"("At Infinity"=TRUE) -> ("New Light Refnum"=w227:refnum<vi>)  [unwired: 2 in, 8 out]
      n82 = property class="SceneLight"(reference=w227, "Direction"=cluster{"X":sgl, "Y":sgl, "Z":sgl} {"X"=0.0, "Y"=0.0, "Z"=10000.0}, "Diffuse Color"=T12 {"Alpha"=1.0, "Blue"=1.0, "Green"=1.0, "Red"=1.0}, "atInfinity"=TRUE ("At Infinity"), "Light Number"=0, "Position"=T11 {"X"=10000.0, "Y"=0.0, "Z"=10000.0}, "Specular Color"=T10 {"Red"=1.0, "Green"=0.0, "Blue"=0.0, "Alpha"=0.0}) -> (reference out=w224:refnum<vi>)  [unwired: 1 in, 1 out]
      n83 = call-poly <vilib>:"Create Object.vi"("Name"="PointCloud Object") -> ("Scene:New Object"=w226:refnum<vi>)  [unwired: 9 in, 1 out]
      n84 = Multiply(x=w217, y=w216) -> (x*y=w218:i32)
      n85 = for {
        N: w218 -> [_]
        tunnel: [w231] -> w215 mode=indexing
        i -> [w231]
        # "indices"
      }
      n86 = invoke class="SceneObject" method="Light.Add Light"(reference=w226, "Light"=w224) -> (reference out=w219:refnum<vi>)  [unwired: 2 in, 3 out]
    }
  }
  n87 = call "rs3_close all.vi"("rscontext"=w35, "queue in"=w40, "error in (no error)"=w39, "device_list"=w36, "Dev in"=w16, "Sensor in"=w27) -> ("Close Error"=→"Close Error":string)  [unwired: 4 in, 1 out]
